vi "Scan Error Handler.vi"(8 "Error In":errorcluster, 11 "HTTP Response":string) -> (0 "Error Out":errorcluster)   [LabVIEW 2019, in "PF_API.lvclass"]
doc: "Formats the error based on the scan response."
uses:
  PF_API.lvclass
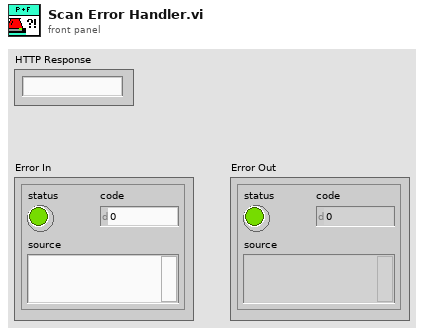
[diagram p1: front panel]
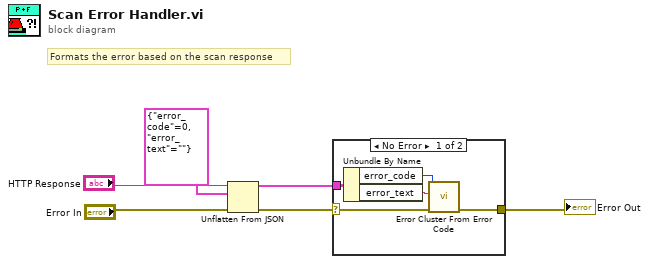
[diagram p0: block diagram]
diagram:
  # "Formats the error based on the scan response"
  n1 = Unflatten From JSON(JSON string="HTTP Response", type and defaults=cluster{"error_code":i32, "error_text":string} {"error_code"=0, "error_text"=""}, error in (no error)="Error In") -> (value=w1:cluster{"error_code":i32, "error_text":string}, error out=w3:errorcluster)  [unwired: 4 in]
  n2 = case shown="No Error" w3 {
    selector: w3 -> [w11 w12]
    tunnel: [w10 w12] -> w2
    tunnel: w1 -> [w9 _]
    frame No Error {
      n3 = Unbundle By Name(w9) -> ("error_code"=w8:i32, "error_text"=w7:string)
      n4 = call <vilib>:"Error Cluster From Error Code.vi"("error in (no error)"=w11, "error message (\"\")"=w7, "error code (0)"=w8) -> ("error out"=w10:errorcluster)  [unwired: 6 in]
    }
    frame Error {
    }
  }
  "Error Out" <- w2
